vi "IIC Slave Write Bytes.vi"(6 "TimeOutMs":i32, 7 "WriteLen":i32, 9 "pWriteData":u8[](array[numeric])=array[20480 elements], 10 "IICIndex":i32, 11 "DevIndex":i32) -> (3 "function return":i32)   [LabVIEW 2010, in "usb2iic.lvlib"]
doc: "int WINAPI IIC_SlaveWriteBytes(int DevIndex,int IICIndex,unsigned char *pWriteData,int WriteLen,int TimeOutMs);"
uses:
  usb2iic.lvlib
  USB2XXX.dll
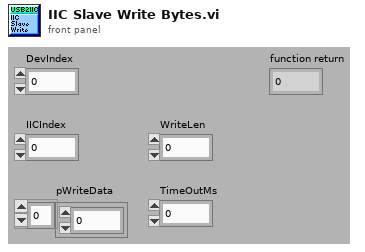
[diagram p1: front panel]
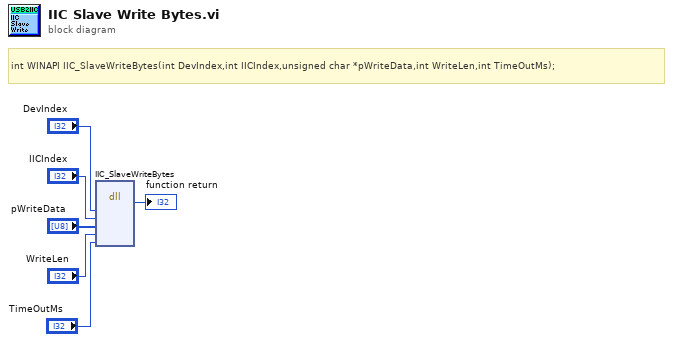
[diagram p0: block diagram]
diagram:
  # "int WINAPI IIC_SlaveWriteBytes(int DevIndex,int IICIndex,unsigned char *pWriteData,int WriteLen,int TimeOutMs);"
  n1 = dll-call lib="G:/OtherWork/USB2XXX_Example/trunk/Labview/PublicFiles/usb2iic/USB2XXX.*" fn="IIC_SlaveWriteBytes"("DevIndex"="DevIndex", "IICIndex"="IICIndex", "pWriteData"="pWriteData", "WriteLen"="WriteLen", "TimeOutMs"="TimeOutMs") -> (→"function return":i32)  [unwired: 8 in, 2 out]
